vi "Convert_to_voltage.vi"(2 "Digital Value":sgl) -> (7 "Voltage Out":sgl)   [LabVIEW 2020]
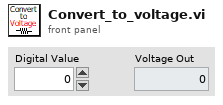
[diagram p1: front panel]
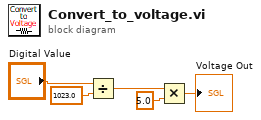
[diagram p0: block diagram]
diagram:
  n1 = Divide(x="Digital Value", y=sgl 1023.0) -> (x/y=w3:sgl)
  n2 = Multiply(x=w3, y=sgl 5.0) -> (x*y=→"Voltage Out":sgl)
